vi "Update String by Index.vi"(6 "Timestamp (Now)":dbl, 8 "error in (no error)":errorcluster, 9 "String":string, 10 "Index":i32, 11 "StringGroup in":refnum<class "Group STR.lvclass">) -> (0 "error out":errorcluster, 3 "StringGroup out":refnum<class "Group STR.lvclass">)   [LabVIEW 2020, in "Vecto.lvlib" / "Group STR.lvclass"]
uses:
  Group STR.lvclass
  C:/dev/lv20CE/relink/lv-vecto/Vecto/Group/Group.lvclass
  Group STR.lvclass/Group STR.ctl
  Group/Group.lvclass
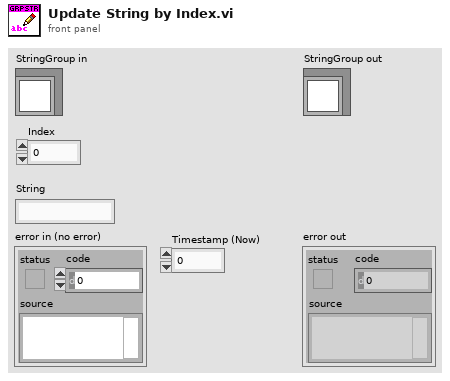
[diagram p1: front panel]
types:
  T1 = typedef "Vecto.lvlib/StringGroup.lvclass/Ref.ctl" = cluster{"Strings":string[], "Timestamp":dbl[]}
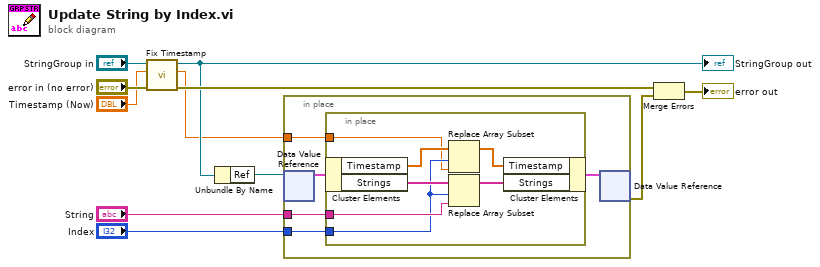
[diagram p0: block diagram]
diagram:
  n1 = call "Fix Timestamp.vi"("error in (no error)"="error in (no error)", "Timestamp in"="Timestamp (Now)", "GroupAbstract in"="StringGroup in") -> ("error out"=w10:errorcluster, "Timestamp"=w3:dbl, "GroupAbstract out"=w6:refnum<class "Group STR.lvclass">)  [unwired: 6 in]
  "StringGroup out" <- w6
  n2 = Unbundle By Name(w6) -> ("Ref"=w7:refnum<data-value>)
  n3 = in-place {
    in-place-border: "Index" -> [w14]
    in-place-border: "String" -> [w13]
    in-place-border: w3 -> [w12]
    n4 = in-place-dvr #1(w7) -> (w16:T1)  [unwired: 1 out]
    n5 = in-place {
      in-place-border: w14 -> [w21]
      in-place-border: w13 -> [w22]
      in-place-border: w12 -> [w19]
      n6 = in-place-cluster #2(w16) -> ("Timestamp"=w20:dbl[], "Strings"=w23:string[])
      n7 = Replace Array Subset(array=w20, new element=w19, index=w21) -> (w17:dbl[])
      n8 = Replace Array Subset(array=w23, new element=w22, index=w21) -> (w18:string[])
      n9 = in-place-cluster #2("Timestamp"=w17, "Strings"=w18) -> (w15:T1)
    }
    n10 = in-place-dvr #1(w15) -> (w1:errorcluster)  [unwired: 1 out]
  }
  n11 = Merge Errors(w10, w1) -> (→"error out":errorcluster)
